vi "e.gate Example - HighSpeedPort Read Buffer.vi"(8 "Fehler (Eingang, kein Fehler)":errorcluster, 11 "IP Address":string) -> (0 "error out":errorcluster)   [LabVIEW 2016]
uses:
  e.gate Protocol Type.ctl
panel:
  out "大小":i32[](array[numeric])
  out "子数组":dbl[](array[numeric]) format="%#.10f"
  in  "MaxFrames":dbl(slide) min=0.0 max=100000.0 scale=0.0..100000.0
  out "Tabellenelement":string[][](table)
  out "IP Address":string
  in  "Channel List":i32(listbox)
  out "Signal":dbl[](graph)
  in  "Stop":bool
  # "EXAMPLE - HighSpeedPort buffer communication"
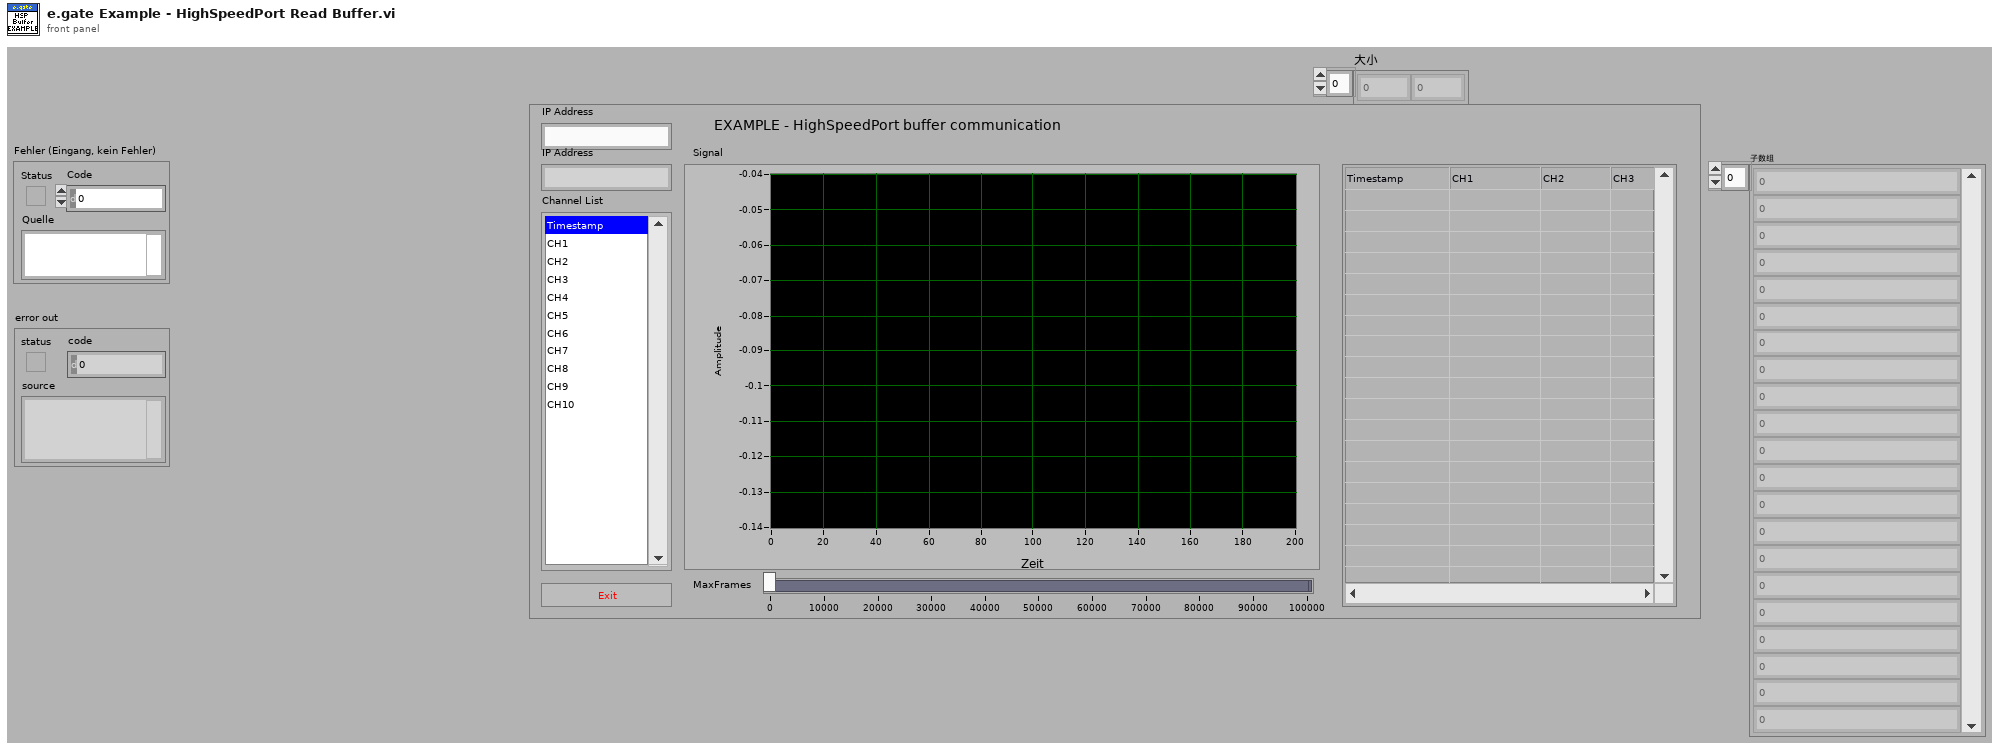
[diagram p1: front panel]
types:
  T1 = typedef "e.gate Protocol Type.ctl" = enum16{"ASCII", "HighspeedPort Online", "HighspeedPort Buffer", "eGateHighspeedPortDLL "}
  T2 = typedef "e.gate Configuration.ctl" = cluster{"connection ID":refnum<k5>, "IPAddress":string, "BufferIndex":i32, "StateMessage":string, "StateCode":i8, "HeaderSize":i32, "BufferSize":i32, "IsBigEndian":i32, "Version":i32, "ChannelCount":i32, "FrameLength":i32, "StartTime":dbl, "dActTimeToSecondFactor":dbl, "StartTimeToDayFactor":dbl, "BufferFillRate":dbl, "SampleRate":dbl, "ChannelData":T3[], "DecodeTimeFormat":string, "SummaryPath":string, "WithCheckSum":i32, "dActTimeDataType":T4, "MaxWriteCount":i32, "MaxReadCount":i32, "TempOffsetRead":i32, "TempLengthRead":i32, "Protocol":T1, "IsSupported":i32, "InputAccessList":i32[], "OutputAccessList":i32[], "DataSource":enum16{"CircleBuffer", "test.con Logger", "test.con Archive"}, "Modules":T5[], "DLL-Handle":T6}
  T3 = typedef "e.gate Channel Data.ctl" = cluster{"VariableName":string, "DataDirection":string, "DataType":string, "DataTypeIndex":T4, "Precision":i16, "FieldLengtht":i16, "ByteCount":i32, "Format":string, "Unit":string, "InputAccessOffset":i32, "OutputAccessOffset":i16, "InputAccessIndex":i16, "OutputAccessIndex":i16, "VarType":string}
  T4 = typedef "e.gate Data Type.ctl" = enum16{"NO", "BOOL", "SINT8", "USINT8", "SINT16", "USINT16", "SINT32", "USINT32", "FLOAT", "SET8", "SET16", "SET32", "DOUBLE", "SINT64", "USINT64", "SET64"}
  T5 = typedef "e.gate Module  Data.ctl" = cluster{"Type":string, "Location":string, "VariablesCount":i16, "UartIndex":i16, "Address":i16, "SystemOffset":i16}
  T6 = typedef "e.gateHSP_DLLhandle.ctl" = cluster{"clientInstance":i32, "connectionInstance":i32}
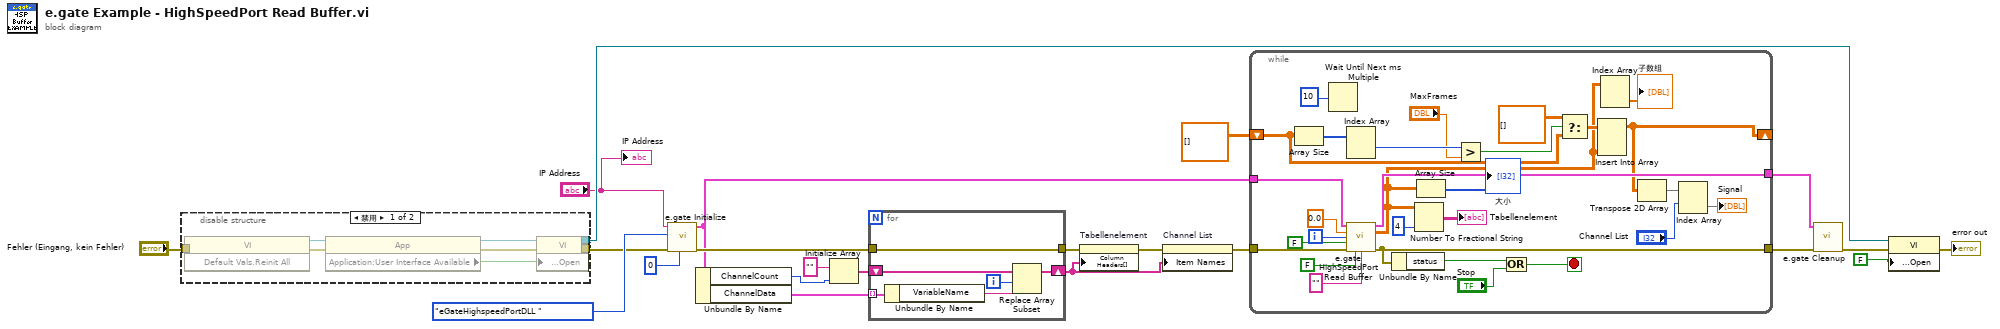
[diagram p0: block diagram]
diagram:
  n1 = disable-structure shown="禁用" {
    disable-tunnel: [w25 _] -> w12
    disable-tunnel: "Fehler (Eingang, kein Fehler)" -> [w24 _]
    disable-tunnel: [w23 _] -> w1
    frame Disabled {
      n2 = invoke class="VI" method="Default Vals.Reinit All"(error in=w24) -> (reference out=w29:refnum<vi>, error out=w27:errorcluster)  [unwired: 2 in, 1 out]
      n3 = property class="App"(error in=w27) -> (error out=w26:errorcluster, "Application:User Interface Available"=w28:bool)  [unwired: 1 in, 1 out]
      n4 = property class="VI"(reference=w29, error in=w26, "Front Panel.Open"=w28) -> (reference out=w25:refnum<vi>, error out=w23:errorcluster)
    }
    frame Enabled {
    }
  }
  n5 = call "e.gate Initialize.vi"("Buffer Index"=0, "error in (no error)"=w1, "Protocol"=e.gate_Protocol_Type."eGateHighspeedPortDLL ", "IP Address"="IP Address") -> ("error out"=w14:errorcluster, "e.gate Configuration"=w9:T2)  [unwired: 6 out]
  n6 = Unbundle By Name(w9) -> ("ChannelCount"=w15:i32, "ChannelData"=w18:T3[])
  n7 = Initialize Array("" ("DecodeTimeFormat"), w15) -> (w16:string[])
  n8 = for {
    tunnel: w18 -> [w33] mode=indexing
    shift-right: [w31] -> w5
    shift-left: w16 -> [w34]
    tunnel: w14 -> [w30]
    tunnel: [w30] -> w7
    i -> [w35]
    n9 = Unbundle By Name(w33) -> ("VariableName"=w32:string)
    n10 = Replace Array Subset(array=w34, new element=w32, index=w35) -> (w31:string[])
  }
  n11 = property on="Tabellenelement" class="Tbl (严格)"(error in=w7, "Column Headers[]"=w5) -> (error out=w6:errorcluster)  [unwired: 1 in, 1 out]
  n12 = property on="Channel List" class="LstBox (严格)"(error in=w6, "Item Names"=w5) -> (error out=w3:errorcluster)  [unwired: 1 in, 1 out]
  n13 = while {
    tunnel: w9 -> [w64]
    tunnel: w3 -> [w63]
    tunnel: [w62] -> w20
    tunnel: [w43] -> w19
    shift-right: [w57] -> _
    shift-left: dbl[][] [] ("Value") -> [w48]
    i -> [w44]
    stop <- w61 stop-if-true
    n14 = Array Size(array=w48) -> (size(s)=w49:i32[])
    n15 = Wait Until Next ms Multiple(millisecond multiple=u32 10 ("Vielfache von ms")) -> ()  [unwired: 1 out]
    n16 = Index Array(array=w49) -> (element #1=w47:i32)  [unwired: 2 in, 1 out]
    n17 = call "e.gate HighSpeedPort Read Buffer.vi"("e.gate Configuration In"=w64, "Backtime"=0.0, "Iteration"=w44, "force Backtime"=FALSE, "error in (no error)"=w63, "No Erasing"=FALSE, "DecodeTimeFormat"="") -> ("e.gate Configuration Out"=w62:T2, "Value"=w37:dbl[][], "error out"=w43:errorcluster)  [unwired: 6 out]
    n18 = Unbundle By Name(w43) -> ("status"=w60:bool)
    n19 = Number To Fractional String(number=w37, precision (6)=i16 4 ("Breite (-)")) -> (F-format string=→"Tabellenelement":string[][])  [unwired: 2 in]
    n20 = Array Size(array=w37) -> (size(s)=→"大小":i32[])
    n21 = Greater?(x=w47, y="MaxFrames") -> (0:w46:bool)
    n22 = Or(x=w60, y="Stop") -> (x .or. y?=w61:bool)
    n23 = Select(t=dbl[][] [], s=w46, f=w48) -> (s? t:f=w55:dbl[][])
    n24 = Insert Into Array(array=w55, new element=w37) -> (w57:dbl[][])  [unwired: 2 in]
    n25 = Index Array(array=w37) -> (element=→"子数组":dbl[])  [unwired: 2 in]
    n26 = Transpose 2D Array(2D array=w57) -> (transposed array=w52:dbl[][])
    n27 = Index Array(array=w52, index (row)="Channel List") -> (element=→"Signal":dbl[])  [unwired: 1 in]
  }
  n28 = call "e.gate Cleanup.vi"("error in (no error)"=w19, "e.gate Configuration"=w20) -> ("error out"=w2:errorcluster)  [unwired: 9 out]
  n29 = property class="VI"(reference=w12, error in=w2, "Front Panel.Open"=FALSE ("Frontpanel-Fenster:Öffnen")) -> (error out=→"error out":errorcluster)  [unwired: 1 out]
  "IP Address" <- "IP Address"
